vi "GetPrivateKey.vi"(0 "e":cluster{"Boolean":bool, "Array":u64[]}, 1 "n":cluster{"Boolean":bool, "Array":u64[]}, 2 "Version":cluster{"Boolean":bool, "Array":u64[]}, 5 "d":cluster{"Boolean":bool, "Array":u64[]}, 7 "p":cluster{"Boolean":bool, "Array":u64[]}, 9 "q":cluster{"Boolean":bool, "Array":u64[]}, 11 "d mod(p - 1)":cluster{"Boolean":bool, "Array":u64[]}, 12 "d mod(q - 1)":cluster{"Boolean":bool, "Array":u64[]}, 13 "q^-1 mod(p)":cluster{"Boolean":bool, "Array":u64[]}) -> (8 "Public Key":string)   [LabVIEW 2023]
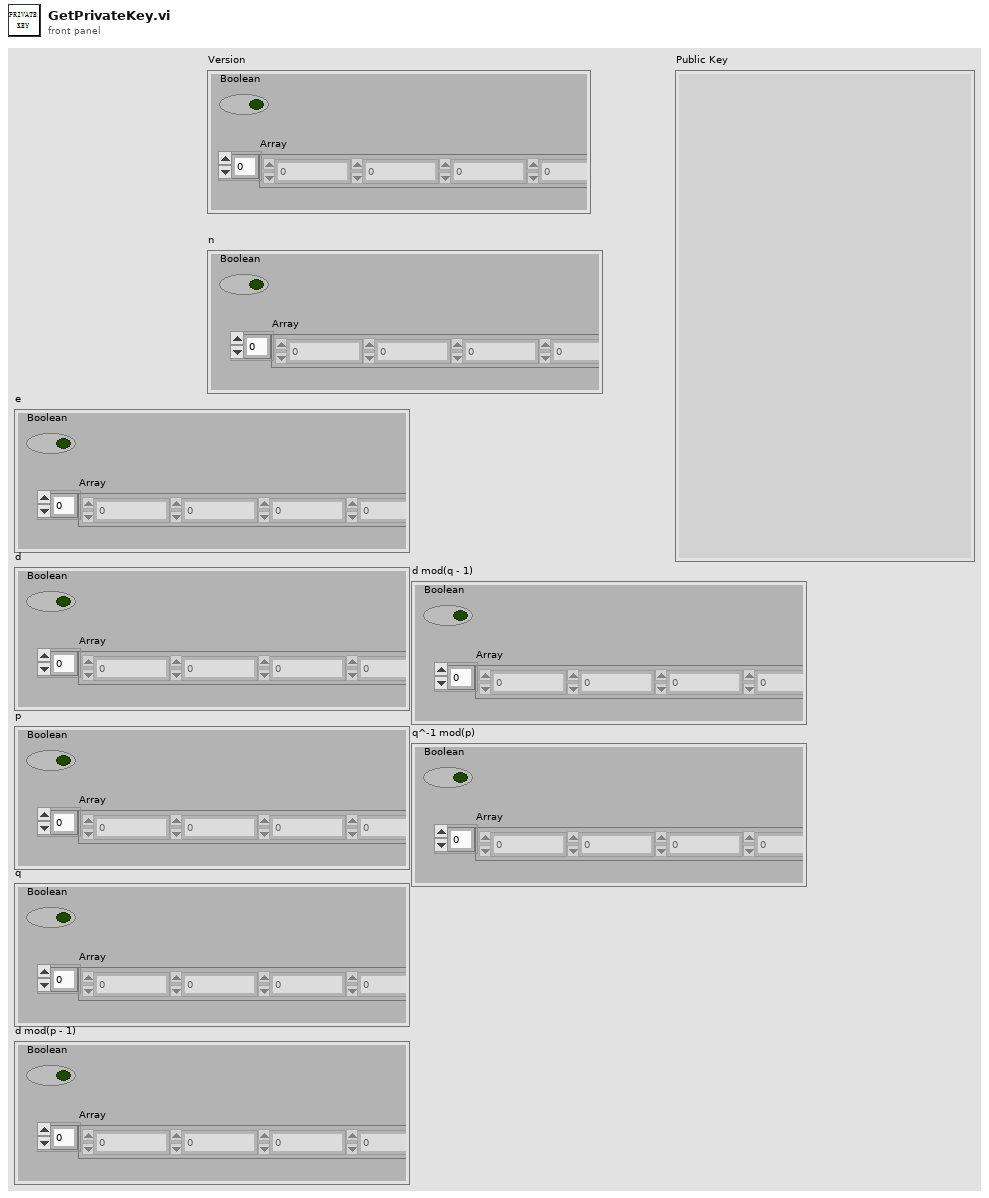
[diagram p1: front panel]
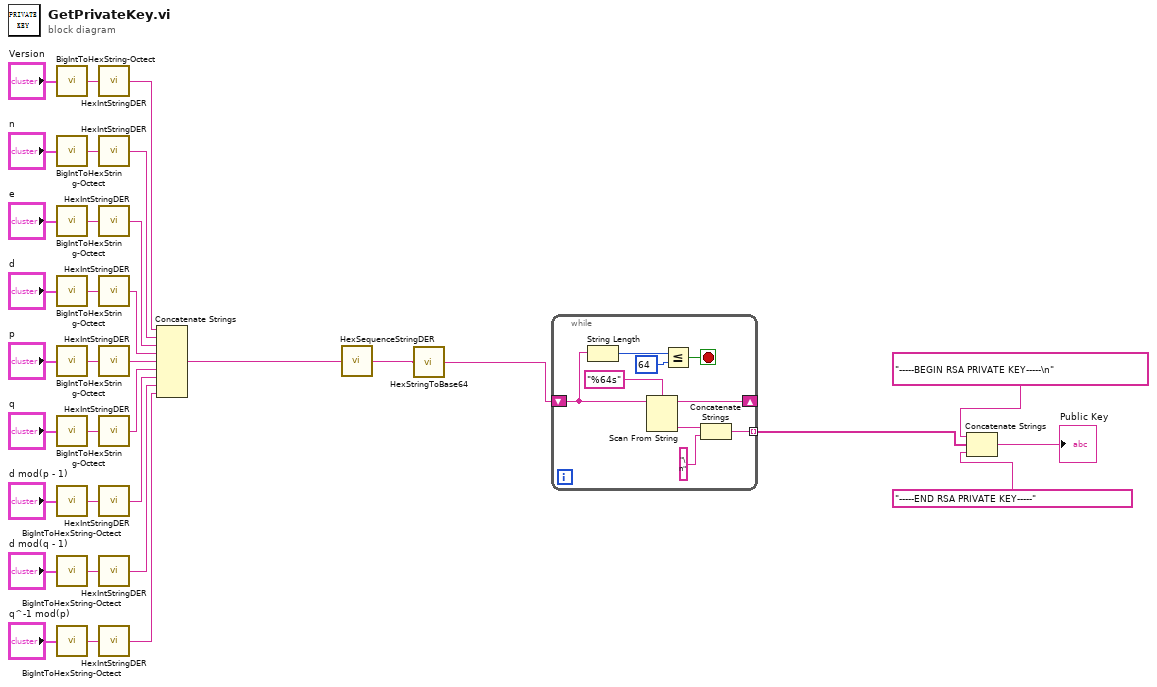
[diagram p0: block diagram]
diagram:
  n1 = call "BigIntToHexString-Octect.vi"("a"="Version") -> ("Hex string"=w34:string)
  n2 = call "BigIntToHexString-Octect.vi"("a"="n") -> ("Hex string"=w33:string)
  n3 = call "BigIntToHexString-Octect.vi"("a"="e") -> ("Hex string"=w21:string)
  n4 = call "BigIntToHexString-Octect.vi"("a"="d") -> ("Hex string"=w19:string)
  n5 = call "BigIntToHexString-Octect.vi"("a"="p") -> ("Hex string"=w17:string)
  n6 = call "BigIntToHexString-Octect.vi"("a"="q") -> ("Hex string"=w15:string)
  n7 = call "BigIntToHexString-Octect.vi"("a"="d mod(p - 1)") -> ("Hex string"=w13:string)
  n8 = call "BigIntToHexString-Octect.vi"("a"="d mod(q - 1)") -> ("Hex string"=w11:string)
  n9 = call "BigIntToHexString-Octect.vi"("a"="q^-1 mod(p)") -> ("Hex string"=w9:string)
  n10 = call "HexIntStringDER.vi"("Hex(formatted integer)"=w34) -> ("DER"=w32:string)
  n11 = call "HexIntStringDER.vi"("Hex(formatted integer)"=w33) -> ("DER"=w31:string)
  n12 = call "HexIntStringDER.vi"("Hex(formatted integer)"=w21) -> ("DER"=w7:string)
  n13 = call "HexIntStringDER.vi"("Hex(formatted integer)"=w19) -> ("DER"=w6:string)
  n14 = call "HexIntStringDER.vi"("Hex(formatted integer)"=w17) -> ("DER"=w5:string)
  n15 = call "HexIntStringDER.vi"("Hex(formatted integer)"=w15) -> ("DER"=w4:string)
  n16 = call "HexIntStringDER.vi"("Hex(formatted integer)"=w13) -> ("DER"=w3:string)
  n17 = call "HexIntStringDER.vi"("Hex(formatted integer)"=w11) -> ("DER"=w2:string)
  n18 = call "HexIntStringDER.vi"("Hex(formatted integer)"=w9) -> ("DER"=w1:string)
  n19 = Concatenate Strings(w32, w31, w7, w6, w5, w4, w3, w2, w1) -> (w30:string)
  n20 = call "HexSequenceStringDER.vi"("Hex(sequence)"=w30) -> ("DER"=w25:string)
  n21 = call "HexStringToBase64.vi"("Hex"=w25) -> ("BASE64 string"=w24:string)
  n22 = while {
    shift-right: [w43] -> _
    shift-left: w24 -> [w38]
    tunnel: [w39] -> w29 mode=indexing
    stop <- w35 stop-if-true
    n23 = String Length(string=w38) -> (length=w37:i32)
    n24 = Scan From String(format string="%64s", input string=w38) -> (remaining string=w43:string, output 1=w40:string)  [unwired: 3 in, 2 out]
    n25 = Less Or Equal?(x=w37, y=64) -> (x <= y?=w35:bool)
    n26 = Concatenate Strings(w40, "\n") -> (w39:string)
  }
  n27 = Concatenate Strings("-----BEGIN RSA PRIVATE KEY-----\n", w29, "-----END RSA PRIVATE KEY-----") -> (→"Public Key":string)
